vi "UART Write Bytes.vi"(7 "Len":u16, 8 "error in (no error)":errorcluster, 9 "pWriteData":string, 10 "UARTIndex":i32, 11 "DevIndex":i32) -> (0 "error out":errorcluster, 3 "function return":i32)   [LabVIEW 2012, in "ControlUART.lvlib"]
doc: "int WINAPI UART_WriteBytes(int DevIndex,int UARTIndex,unsigned char* pWriteData,unsigned short Len);"
uses:
  ControlUART.lvlib
  Ginkgo_Driver.dll
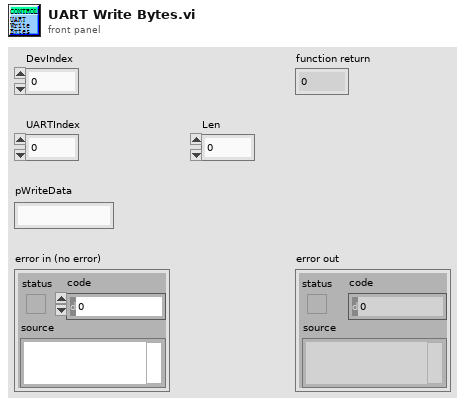
[diagram p1: front panel]
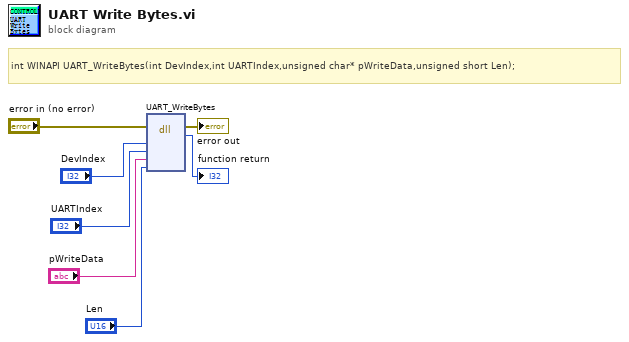
[diagram p0: block diagram]
diagram:
  # "int WINAPI UART_WriteBytes(int DevIndex,int UARTIndex,unsigned char* pWriteData,unsigned short Len);"
  n1 = dll-call lib="E:/Project/vt_ginkgo/truck/Ginkgo Driver/vs2010/Ginkgo_USB-I2C_API_v2.0.3.0/lib/labview_64bit/ControlUART/Ginkgo_Driver.*" fn="UART_WriteBytes"(error in="error in (no error)", "DevIndex"="DevIndex", "UARTIndex"="UARTIndex", "pWriteData"="pWriteData", "Len"="Len") -> (error out=→"error out":errorcluster, →"function return":i32)  [unwired: 6 in, 1 out]
